vi "DL-SMART-MS-Modify-05-02 - 3.0.vi"() -> ()   [LabVIEW 2013]
uses:
  <vilib>/Utility/file.llb/Read From Spreadsheet File (DBL).vi
  <vilib>/vision/driver/NI_Vision_Acquisition_Software.lvlib
panel:
  out "Mass Spectrum (质谱图)":dbl[](graph)
  out "Image":T1(plugin-control)
  in  "Laser parameter":T3
  in  "ADC parameter":T4
  in  "ShutDownSystem":bool
  out "TenAccumulate":cluster{"MassX":dbl[], "TenScans":sgl[]}
  in  "ADC reference":refnum<vi>
  in  "set laser":bool
  in  "SetLaserEnergy":dbl(slide) min=0.0 max=50.0 scale=0.0..20.0
  in  "LaserHV":u8=50 min=1 max=100
  in  "LaserQuantity":u16
  in  "频率/Hz":u8=60
  out "plat zeroed":bool
  out "ADC aquiring":bool
  out "motor moving":bool
  out "busy":bool
  out "Pul.HV-Real":dbl
  in  "ReportResult":bool
  out "Identify Spcetrum":cluster{"all rows":dbl[], "all rows":dbl[]}[](graph)=[{"all rows"=array[50131 elements], "all rows"=array[50131 elements]}, {"all rows"=array[360 elements], "all rows"=[0.0, -15.85746, 0.0, 0.0, -4.11823, 0.0, 0.0, -20.55303, 0.0, 0.0, -3.65583, 0.0, 0.0, -2.69345, 0.0, 0.0, -4.4706, 0.0, 0.0, -6.07537, 0.0, 0.0, -4.25015, 0.0, 0.0, -6.95758, 0.0, 0.0, -2.04252, 0.0, 0.0, -7.70754, 0.0, 0.0, -4.28864, 0.0, 0.0, -4.00869, 0.0, 0.0, -4.47517, 0.0, 0.0, -14.21368, 0.0, 0.0, -6.66072, 0.0, 0.0, -6.50078, 0.0, 0.0, -3.75903, 0.0, 0.0, -17.29715, 0.0, 0.0, -6.92254, 0.0, 0.0, -2.52353, 0.0, 0.0, -3.06405, 0.0, 0.0, -16.54211, 0.0, 0.0, -5.10076, 0.0, 0.0, -8.01669, 0.0, 0.0, -40.71695, 0.0, 0.0, -4.03763, 0.0, 0.0, -3.14159, 0.0, 0.0, -2.79298, 0.0, 0.0, -13.41979, 0.0, 0.0, -7.6464, 0.0, 0.0, -6.18956, 0.0, 0.0, -2.44901, 0.0, 0.0, -5.1704, 0.0, 0.0, -3.62455, 0.0, 0.0, -6.443, 0.0, 0.0, -24.18432, 0.0, 0.0, -37.78631, 0.0, 0.0, -4.28528, 0.0, 0.0, -3.21654, 0.0, 0.0, -3.13522, 0.0, 0.0, -4.8477, 0.0, 0.0, -3.80614, 0.0, 0.0, -8.10386, 0.0, 0.0, -2.86382, 0.0, 0.0, -17.8978, 0.0, 0.0, -4.74503, 0.0, 0.0, -9.4855, 0.0, 0.0, -5.75364, 0.0, 0.0, -80.29859, 0.0, 0.0, -5.18928, 0.0, 0.0, -28.13783, 0.0, 0.0, -6.84449, 0.0, 0.0, -4.07742, 0.0, 0.0, -2.99391, 0.0, 0.0, -4.60838, 0.0, 0.0, -3.257, 0.0, 0.0, -5.79015, 0.0, 0.0, -24.98325, 0.0, 0.0, -4.30828, 0.0, 0.0, -5.54625, 0.0, 0.0, -5.47663, 0.0, 0.0, -100.0001, 0.0, 0.0, -21.11295, 0.0, 0.0, -12.03347, 0.0, 0.0, -6.35092, 0.0, 0.0, -4.71483, 0.0, 0.0, -6.58836, 0.0, 0.0, -3.41548, 0.0, 0.0, -3.10072, 0.0, 0.0, -4.79955, 0.0, 0.0, -4.88109, 0.0, 0.0, -32.02295, 0.0, 0.0, -20.17071, 0.0, 0.0, -9.63953, 0.0, 0.0, -8.63946, 0.0, 0.0, -6.018, 0.0, 0.0, -6.3389, 0.0, 0.0, -14.67808, 0.0, 0.0, -6.22948, 0.0, 0.0, -4.9166, 0.0, 0.0, -44.64096, 0.0, 0.0, -5.6163, 0.0, 0.0, -8.56872, 0.0, 0.0, -11.1186, 0.0, 0.0, -4.42493, 0.0, 0.0, -15.45284, 0.0, 0.0, -2.99091, 0.0, 0.0, -18.05376, 0.0, 0.0, -3.06669, 0.0, 0.0, -35.88844, 0.0, 0.0, -19.12645, 0.0, 0.0, -3.20878, 0.0, 0.0, -2.61247, 0.0, 0.0, -7.79975, 0.0, 0.0, -5.8874, 0.0, 0.0, -5.7487, 0.0, 0.0, -5.43834, 0.0, 0.0, -21.69908, 0.0, 0.0, -64.96584, 0.0, 0.0, -5.77762, 0.0, 0.0, -5.55465, 0.0, 0.0, -4.62119, 0.0, 0.0, -3.61176, 0.0, 0.0, -6.99332, 0.0, 0.0, -4.34549, 0.0, 0.0, -15.09003, 0.0, 0.0, -6.25437, 0.0, 0.0, -21.85243, 0.0, 0.0, -13.24381, 0.0, 0.0, -3.94672, 0.0, 0.0, -3.90192, 0.0, 0.0, -11.14967, 0.0, 0.0, -83.69183, 0.0, 0.0, -11.19559, 0.0, 0.0, -7.83445, 0.0, 0.0, -3.14763, 0.0, 0.0, -6.44728, 0.0, 0.0, -5.69155, 0.0, 0.0, -4.00216, 0.0]}]
  in  "IdentifyMS":bool
  in  "Identification Record (鉴定记录表)":i32(listbox)=6
  in  "Identification Results (单靶鉴定结果)":i32(listbox)=2
  in  "HVEnable":bool
  out "执行进度栏":u8(slide) caption="Vaccum" scale=0.0..1.0
  out "GateClose":bool
  out "LaserOK":bool
  out "HV-OK":bool
  out "Vacuum-OK":bool
  in  "Tab Control":T5(tab)
  in  "Shots":i32
  in  "EditAutoTar":bool
  in  "SinglePoint":bool
  in  "MultiPoints":bool
  in  "MultiTargets":bool
  in  "MCPHV-Set":dbl=1600.0 min=0.0 max=1600.0
  in  "LensHV-Set":dbl=8000.0 min=0.0 max=10000.0
  in  "Tar.HV-Set":dbl=18010.0 min=0.0 max=20000.0
  in  "Pul.HV-Set":dbl=1400.0 min=0.0 max=2000.0
  in  "PulseDelay":dbl
  in  "ADCFreq":dbl
  in  "CH1_Coupling":u64(ring)=2 items=["Volt DC"=1, "Volt AC"=2, "Ampere DC"=4, "Ampere AC"=8, "Ohm"=16]
  in  "Channel 1_Range":dbl(ring)=4.0 items=["80 V"=80.0, "40 V"=40.0, "20 V"=20.0, "8 V"=8.0, "4 V"=4.0, "2 V"=2.0, "800 mV"=0.8, "400 mV"=0.4, "200 mV"=0.2]
  in  "Anal. Setting File":string="High Mass"
  in  "SettingFileSave":bool caption="TakeMS"
  in  "SettingFileAppl":bool caption="TakeMS"
  in  "SettingDel":bool caption="TakeMS"
  in  "RunADC":bool caption="TakeMS"
  out "ADCstatus":bool
  in  "Vac_Prot.":bool
  in  "Turbo_Fore":bool
  in  "Main_Samp":bool
  in  "Samp_Atmos":bool
  in  "Fore_Samp":bool
  in  "StartPump":bool
  in  "SopPump":bool
  in  "Startsystem":bool
  out "TurboSpeed":dbl(knob) scale=0.0..100.0
  out "PumpKW":dbl
  out "PumpAmps":dbl
  out "PumpTemp":u16
  out "PumpVolts":dbl
  in  "laser OFF":bool
  in  "laser ON":bool
  out "cluster":T6
  in  "chamber in":bool caption="TakeMS"
  in  "GO":bool
  in  "Y":dbl min=0.0 max=55.0
  in  "X":dbl min=0.0 max=55.0
  in  "Y+":bool
  in  "Y-":bool
  in  "X-":bool
  in  "X+":bool
  in  "Plat_To_Zero":bool caption="TakeMS"
  in  "Plat_Cal":bool caption="TakeMS"
  out "Ty":dbl
  out "Tx":dbl
  out "Y当前":dbl
  out "X当前":dbl
  out "移动":bool
  out "Y满":bool
  out "Y标":bool
  out "X满":bool
  out "Y0":bool
  out "X0":bool
  out "靶位In/Out":bool
  out "仓门":bool
  out "Y过热":bool
  out "X过热":bool
  out "通讯":bool
  in  "chamber out":bool caption="TakeMS"
  in  "Operation Record":i32(listbox)
  in  "OptionRecordLoad 2":bool caption="TakeMS"
  in  "OptionRecordClear":bool caption="TakeMS"
  in  "OpenCloseGate":bool
  out "Tar.HV-Real":dbl
  out "LensHV-Real":dbl
  out "MCPHV-Real":dbl
  out "Lvaccum":dbl=0.83 format="%#_6e"
  out "Hvaccum":dbl=3.4e-05 format="%#_6e"
  in  "H12":bool
  in  "G12":bool
  in  "F12":bool
  in  "E12":bool
  in  "D12":bool
  in  "C12":bool
  in  "B12":bool
  in  "A12":bool
  in  "H11":bool
  in  "G11":bool
  in  "F11":bool
  in  "E11":bool
  in  "D11":bool
  in  "C11":bool
  in  "B11":bool
  in  "A11":bool
  in  "H10":bool
  in  "G10":bool
  in  "F10":bool
  in  "E10":bool
  in  "D10":bool
  in  "C10":bool
  in  "B10":bool
  in  "A10":bool
  in  "H9":bool
  in  "G9":bool
  in  "F9":bool
  in  "E9":bool
  in  "D9":bool
  in  "C9":bool
  in  "B9":bool
  in  "A9":bool
  in  "H8":bool
  in  "G8":bool
  in  "F8":bool
  in  "E8":bool
  in  "D8":bool
  in  "C8":bool
  in  "B8":bool
  in  "A8":bool
  in  "H7":bool
  in  "G7":bool
  in  "F7":bool
  in  "E7":bool
  in  "D7":bool
  in  "C7":bool
  in  "B7":bool
  in  "A7":bool
  in  "H6":bool
  in  "G6":bool
  in  "F6":bool
  in  "E6":bool
  in  "D6":bool
  in  "C6":bool
  in  "B6":bool
  in  "A6":bool
  in  "H5":bool
  in  "G5":bool
  in  "F5":bool
  in  "E5":bool
  in  "D5":bool
  in  "C5":bool
  in  "B5":bool
  in  "A5":bool
  in  "H4":bool
  in  "G4":bool
  in  "F4":bool
  in  "E4":bool
  in  "D4":bool
  in  "C4":bool
  in  "B4":bool
  in  "A4":bool
  in  "H3":bool
  in  "G3":bool
  in  "F3":bool
  in  "E3":bool
  in  "D3":bool
  in  "C3":bool
  in  "B3":bool
  in  "A3":bool
  in  "H2":bool
  in  "G2":bool
  in  "F2":bool
  in  "E2":bool
  in  "D2":bool
  in  "C2":bool
  in  "B2":bool
  in  "A2":bool
  in  "H1":bool
  in  "G1":bool
  in  "F1":bool
  in  "E1":bool
  in  "D1":bool
  in  "C1":bool
  in  "B1":bool
  in  "A1":bool
  in  "Clear":bool caption="TakeMS"
  in  "Add":bool caption="TakeMS"
  in  "TakeMS-Stop":bool caption="TakeMS"
  in  "TakeMS-Run":bool caption="TakeMS"
  # "Camera (摄像头)"
  # "Laser (激光)"
  # "Acq.(采谱)"
  # "1"
  # "2"
  # "3"
  # "4"
  # "5"
  # "6"
  # "7"
  # "8"
  # "9"
  # "10"
  # "11"
  # "12"
  # "Vacuum(真空)"
  # "A"
  # "Pa"
  # "High"
  # "B"
  # "Low"
  # "Pa"
  # "C"
  # "H.V.(高压)"
  # "D"
  # "Ident. (鉴定图)"
  # "MCP"
  # "V"
  # "E"
  # "Tar."
  # "V"
  # "F"
  # "Pul."
  # "V"
  # "G"
  # "Lens"
  # "V"
  # "H"
  # "Vauum (真空)"
  # "H.V. (高压)"
  # "Laser (激光)"
  # "Gate (仓门)"
  # "SinglePoint (单点)"
  # "MultiPoints (多点)"
  # "MultiTar. (多靶)"
  # "H.V. (高压参数)"
  # "ADC(采集卡设置)"
  # "ADCFreq(采样)"
  # "MCP (探测器)"
  # "V"
  # "Hz"
  # "Tar. (靶)"
  # "V"
  # "Setting File(设置文件)"
  # "Coupling"
  # "Pulse (脉冲)"
  # "V"
  # "IntRange"
  # "V"
  # "Lens (透镜)"
  # "Delay (延时)"
  # "ns"
  # "Turbo Pump"
  # "Sole. Valves"
  # "自锁保护"
  # "机械/分子"
  # "主仓/样仓"
  # "样仓/大气"
  # "机械/样仓"
  # "激光器状态"
  # "mm"
  # "mm"
  # "mm"
  # "mm"
  # "度"
  # "度"
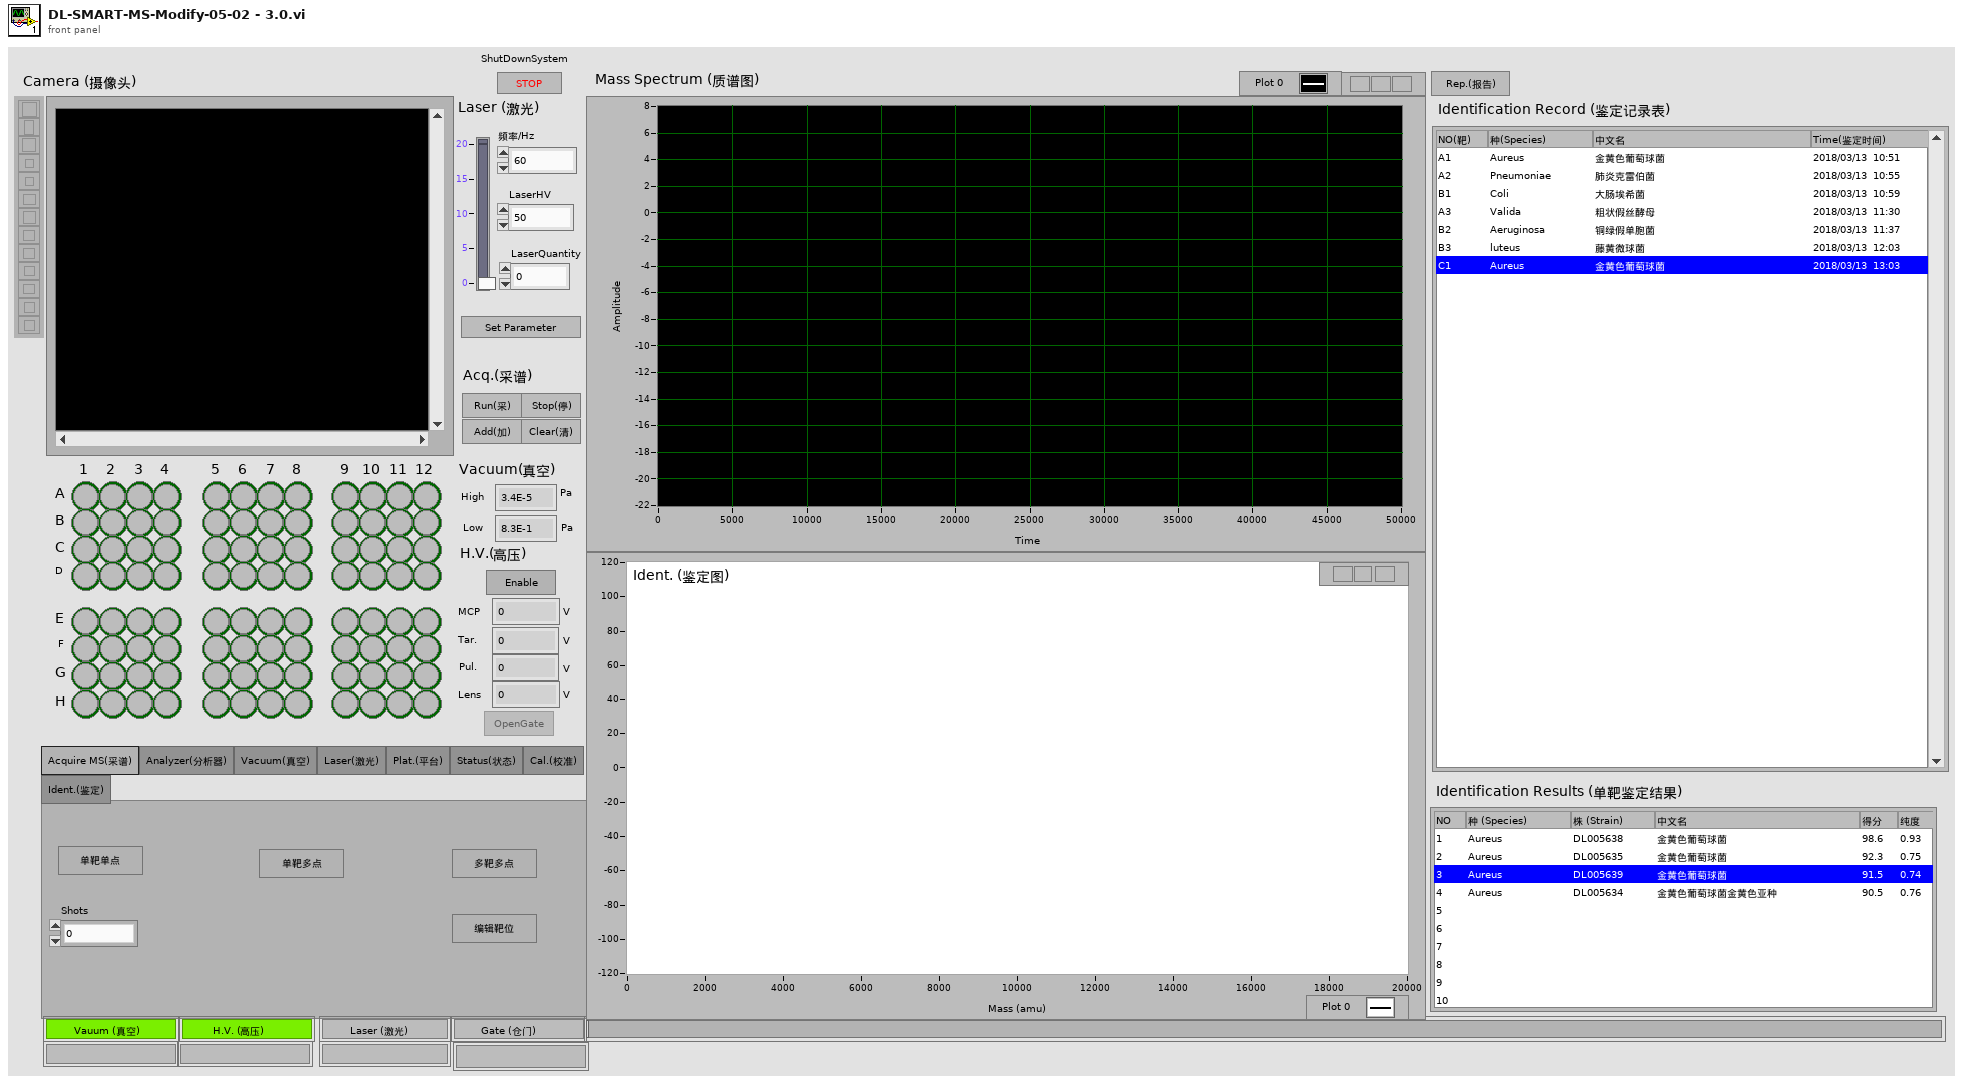
[diagram p1: front panel]
types:
  T1 = typedef "IMAQ Image.ctl" = refnum<image>
  T2 = typedef "Semaphore RefNum" = refnum<k1>
  T3 = cluster{"VISA resource name":refnum<visa-resource-name>, "standby":bool, "semaphore in":T2, "SetLaserEnergy":dbl}
  T4 = cluster{"TpDeviceHandle_t":u32, "Record Length/Samples":u64, "ShotsPerPoint":u16}
  T5 = enum32{"Acquire MS(采谱)", "Analyzer(分析器)", "Vacuum(真空)", "Laser(激光)", "Plat.(平台)", "Status(状态)", "Cal.(校准)", "Ident.(鉴定)"}
  T6 = cluster{"链接":bool, "待机":bool, "发射":bool, "[3]":bool, "内存":bool, "测能":bool, "温警":bool, "静态":bool, "操作":bool}
  T7 = cluster{"laser semaphore":T2, "pump semaphore":T2}
  T8 = enum8{"Enabled", "Disabled", "Disabled and Grayed Out"}
  T9 = cluster{"monitor":refnum<user-event>, "motor status":refnum<user-event>, "motor":refnum<user-event>, "notifier out":refnum<notifier>, "queue out":refnum<queue>, "AI":T2, "DI":T2, "CX":T2, "CY":T2}
  T10 = cluster{"AI Task":refnum<k21>, "AO Task":refnum<k21>, "DO Task":refnum<k21>, "DI Task":refnum<k21>, "PWM x":refnum<k21>, "PWM y":refnum<k21>, "counter x":refnum<k21>, "counter y":refnum<k21>}
  T11 = cluster{"tasks":cluster{"AI Task":refnum<k21>, "AO Task":refnum<k21>, "DO Task":refnum<k21>, "DI Task":refnum<k21>, "PWM x":refnum<k21>, "PWM y":refnum<k21>, "counter x":refnum<k21>, "counter y":refnum<k21>}, "interface":cluster{"monitor":refnum<user-event>, "motor status":refnum<user-event>, "motor":refnum<user-event>, "notifier out":refnum<notifier>, "queue out":refnum<queue>, "AI":T2, "DI":T2, "CX":T2, "CY":T2}, "error out":errorcluster}
  T12 = cluster{"ConfiguredPumpCom":refnum<visa-resource-name>, "ConfiguredLaserCom":refnum<visa-resource-name>}
  T13 = cluster{"Type":u32, "Version":u32, "Flags":u32, "SerialNumberHigh":u32, "SerialNumberLow":u32, "BusType":u32, "InterfaceName":string, "VendorName":string, "ModelName":string, "CameraFileName":string, "CameraAttributeURL":string}[]
  T14 = cluster{"Type":u32, "Version":u32, "Flags":u32, "SerialNumberHigh":u32, "SerialNumberLow":u32, "BusType":u32, "InterfaceName":string, "VendorName":string, "ModelName":string, "CameraFileName":string, "CameraAttributeURL":string}
  T15 = typedef "IMAQdx.ctl" = refnum<k21>
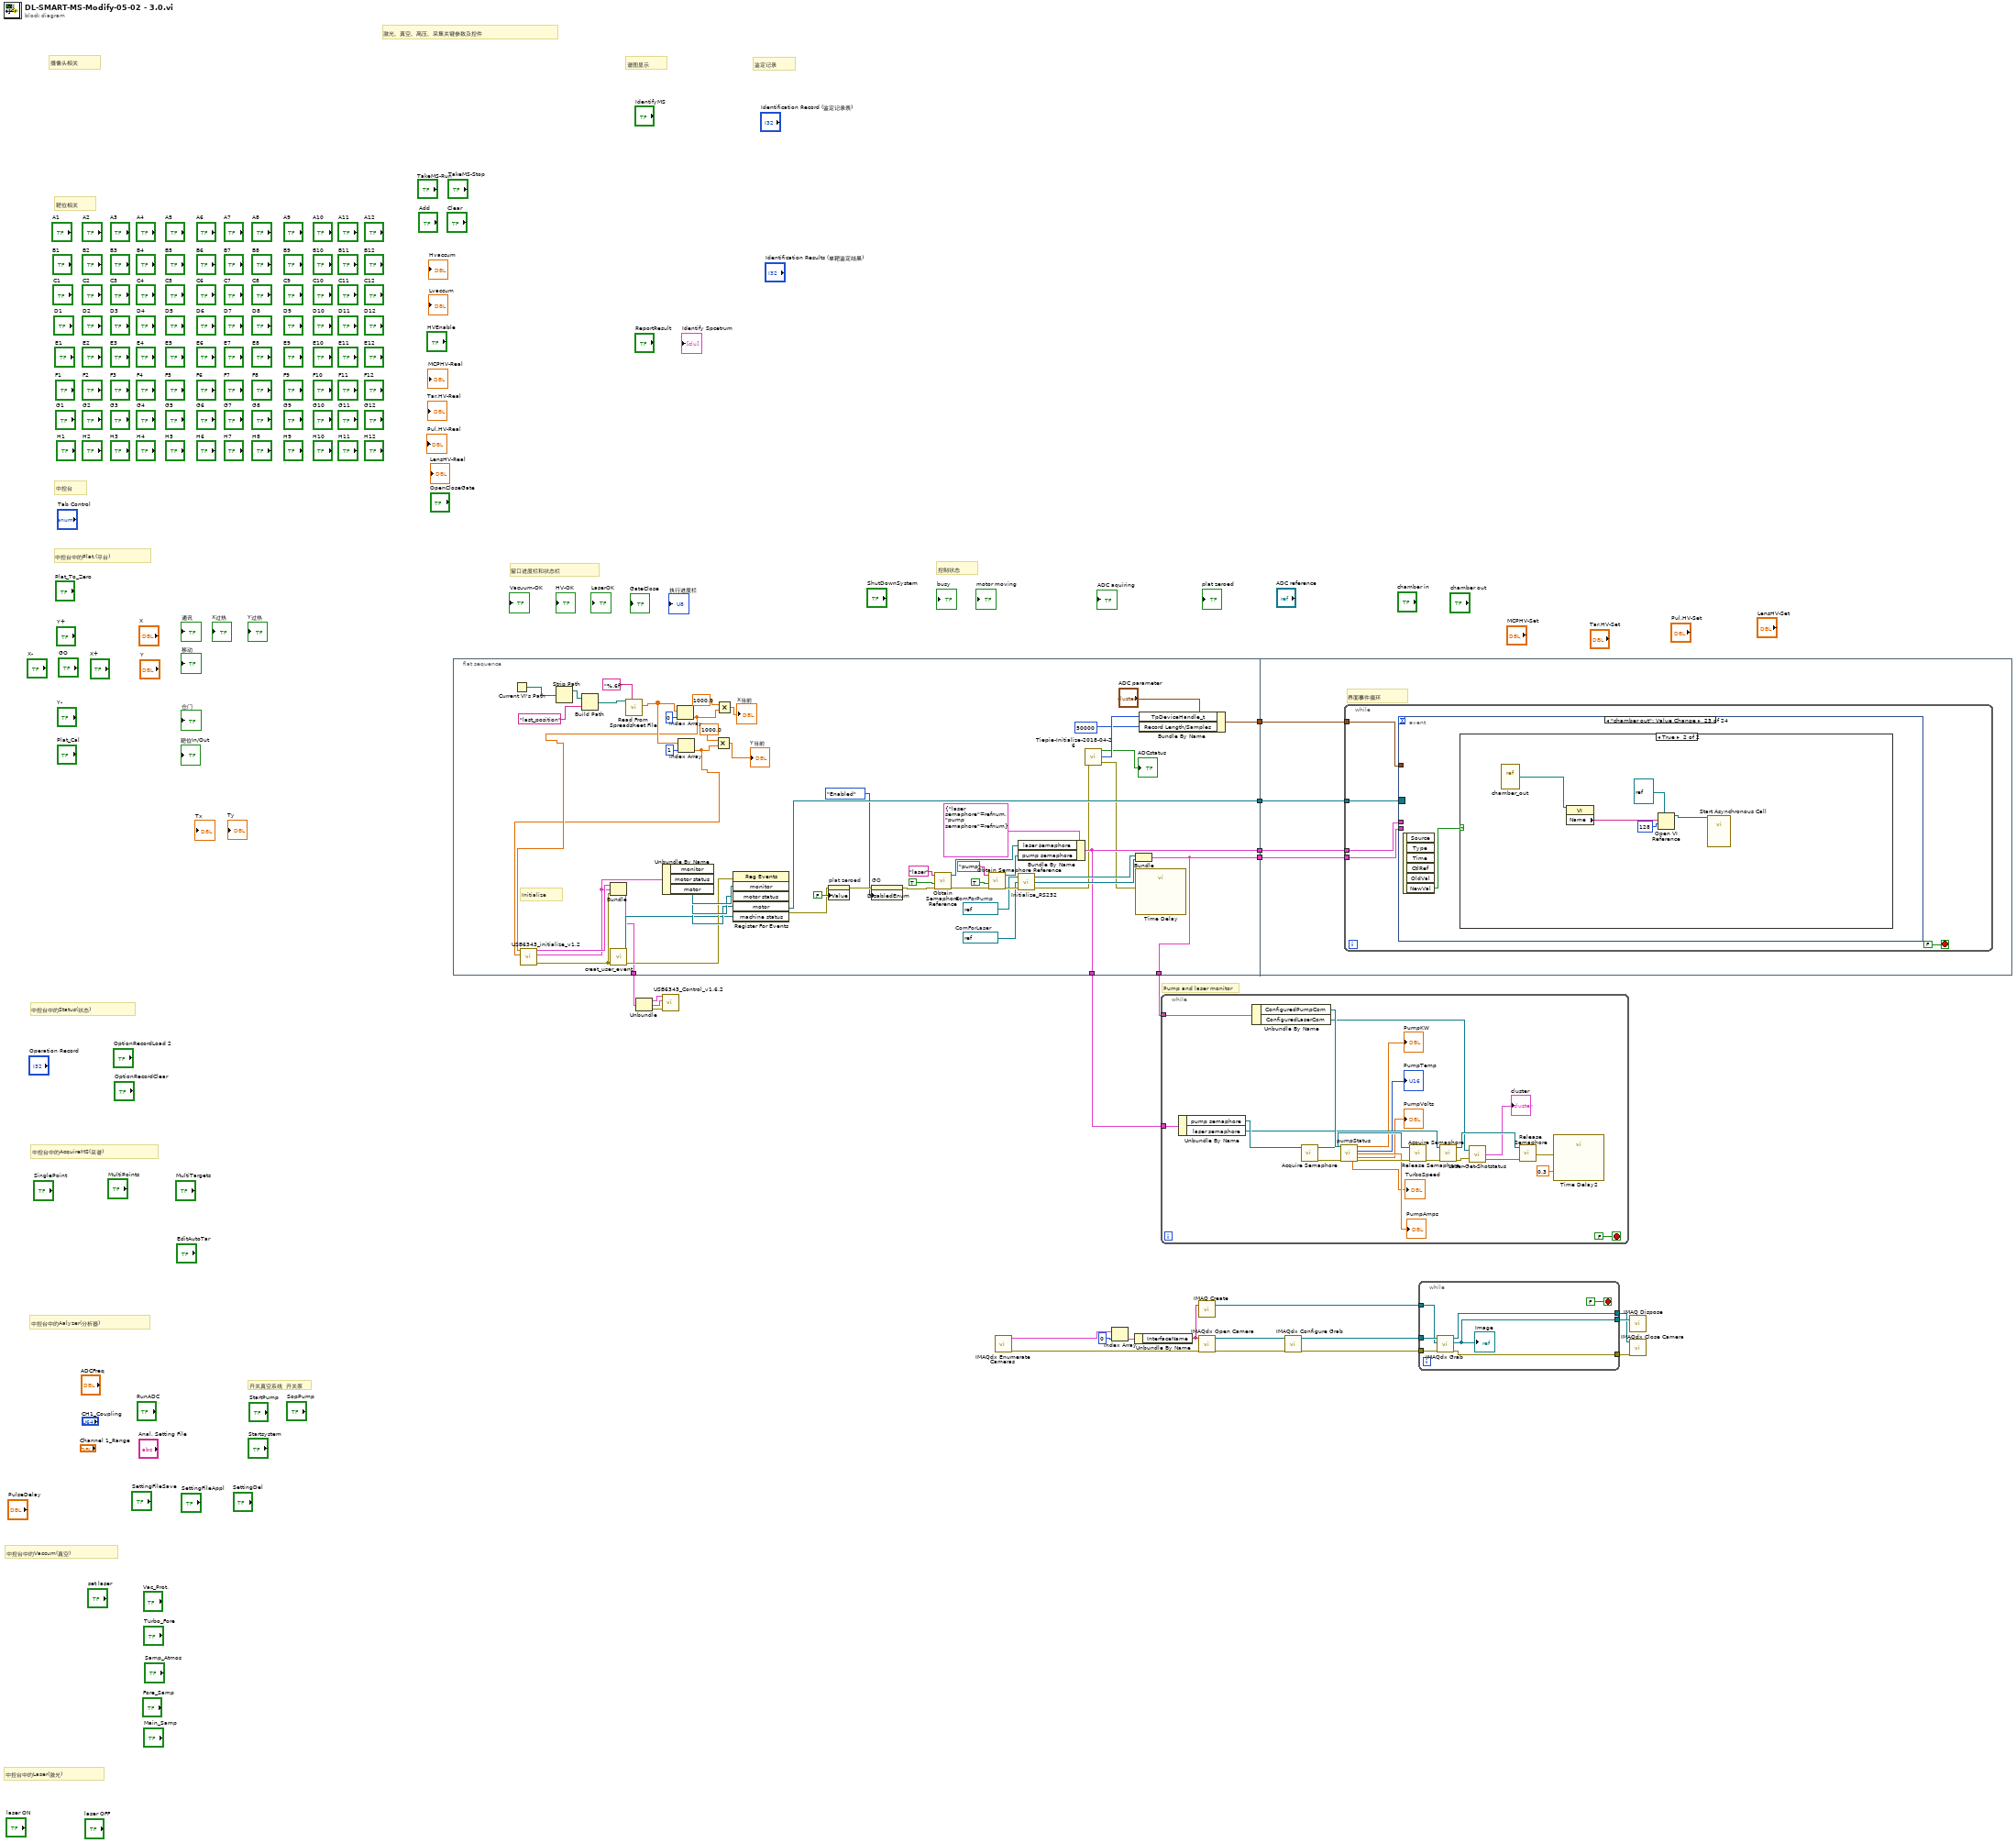
[diagram p0: block diagram]
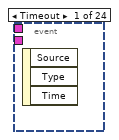
[diagram p2: hidden frame]
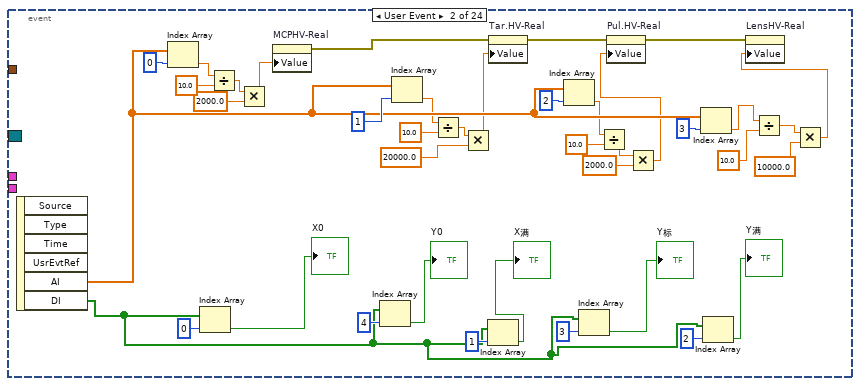
[diagram p3: hidden frame]
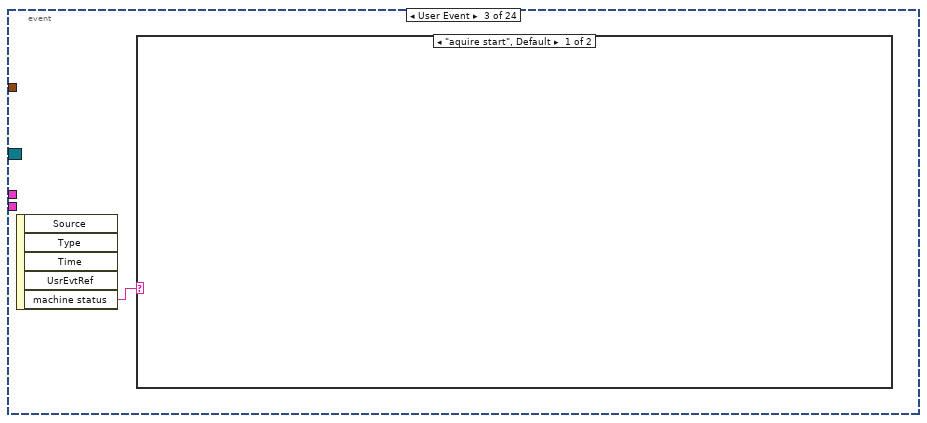
[diagram p4: hidden frame]
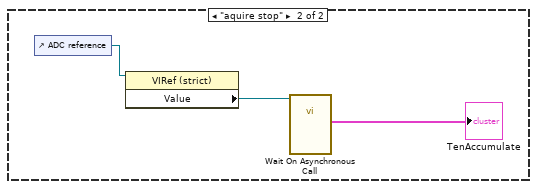
[diagram p5: hidden frame]
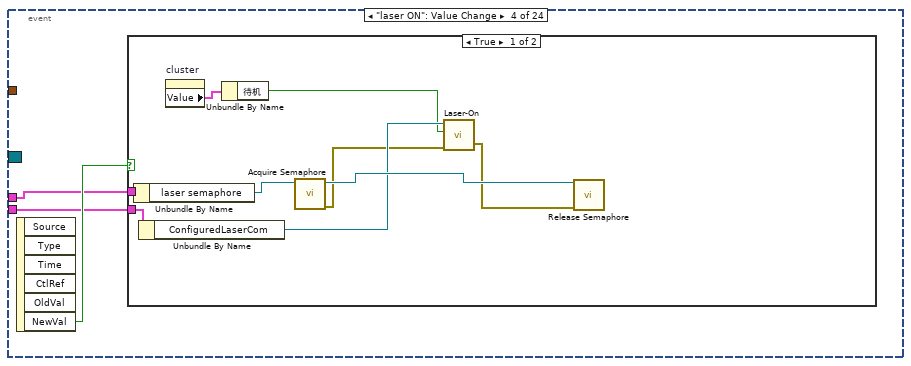
[diagram p6: hidden frame]
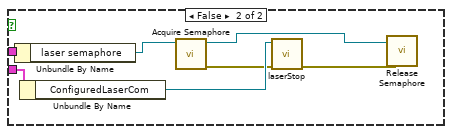
[diagram p7: hidden frame]
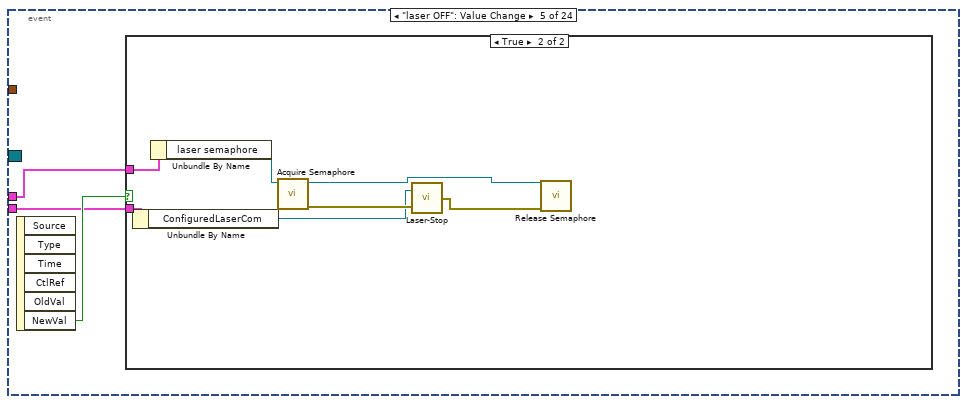
[diagram p8: hidden frame]
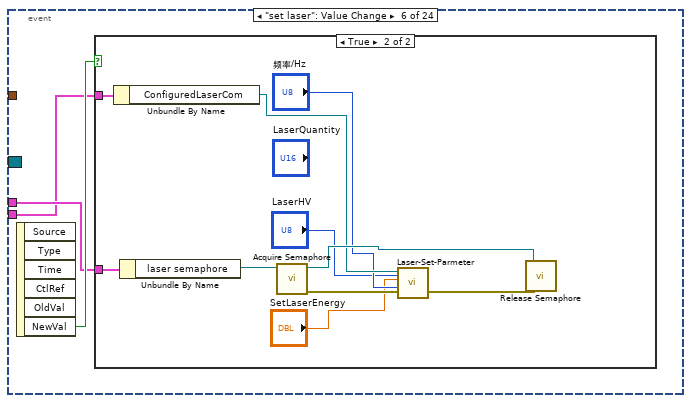
[diagram p10: hidden frame]
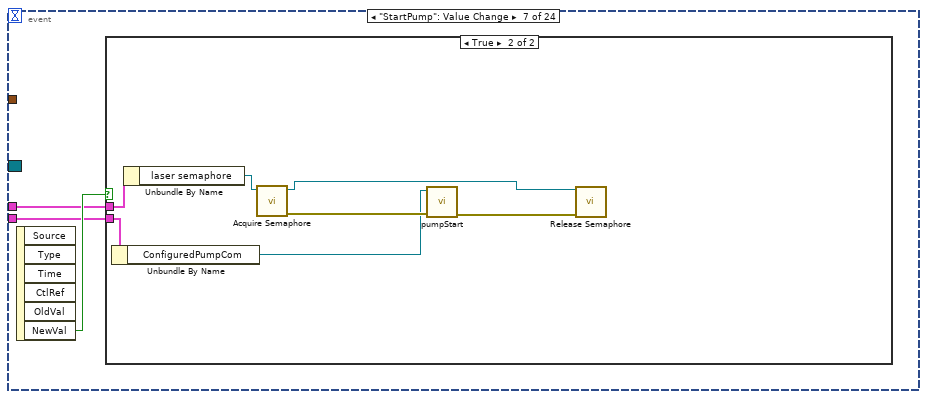
[diagram p12: hidden frame]
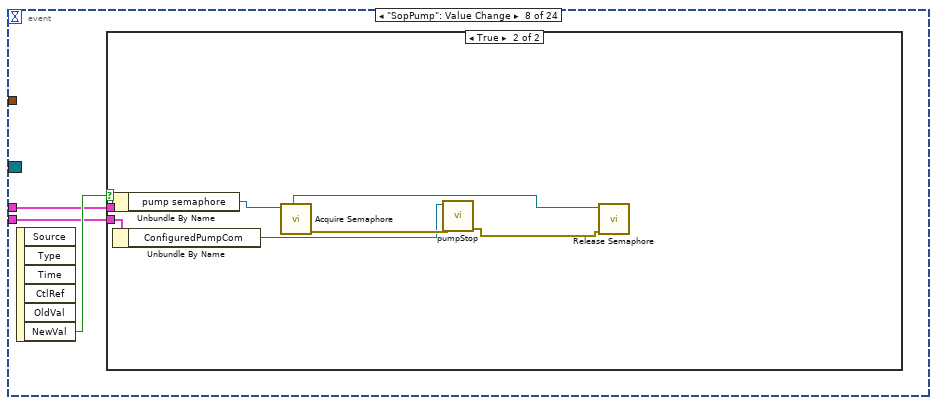
[diagram p14: hidden frame]
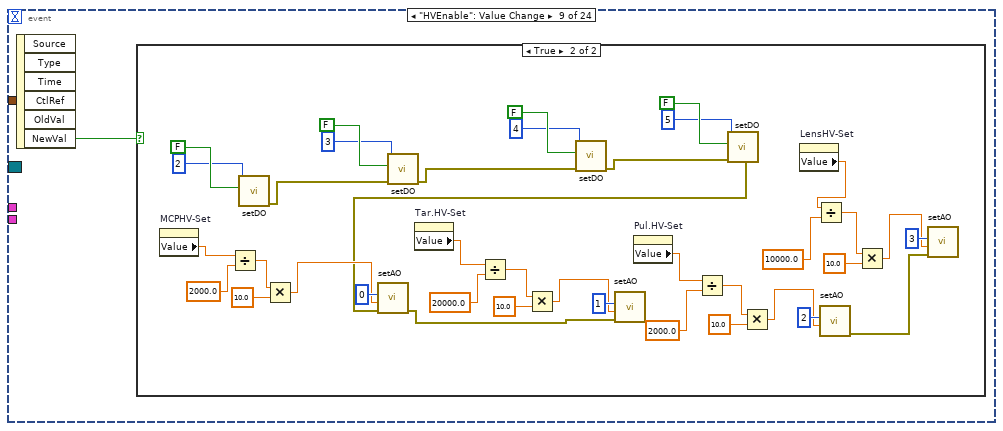
[diagram p16: hidden frame]
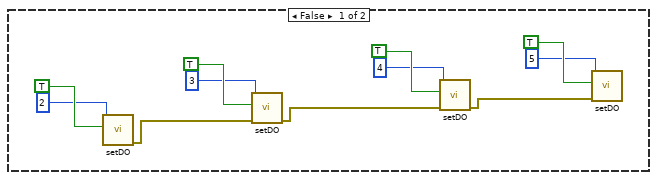
[diagram p17: hidden frame]
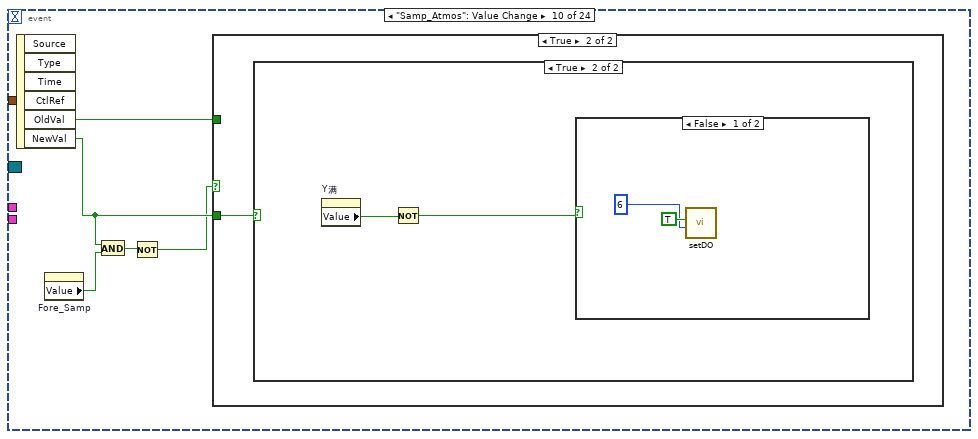
[diagram p18: hidden frame]
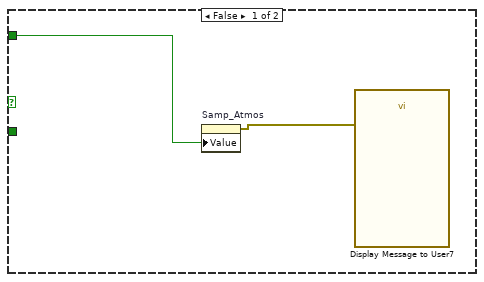
[diagram p19: hidden frame]
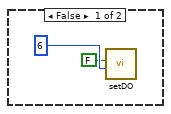
[diagram p20: hidden frame]
diagram:
  # "Pump and laser monitor"
  # "开关真空系统  开关泵"
  # "控制状态"
  # "鉴定记录"
  # "谱图显示"
  # "激光、真空、高压、采集关键参数及控件"
  # "窗口进度栏和状态栏"
  # "中控台中的Laser(激光)"
  # "中控台中的Vaccum(真空)"
  # "中控台中的Aalyzer(分析器)"
  # "中控台中的AcquireMS(采谱)"
  # "中控台中的Status(状态)"
  # "中控台中的Plat.(平台)"
  # "中控台"
  # "靶位相关"
  # "摄像头相关"
  n1 = flat-sequence {
    tunnel: [w71] -> w23
    tunnel: [w48] -> w22
    tunnel: [w48] -> w20
    tunnel: [w47] -> w21
    tunnel: [w47] -> w19
    tunnel: [w51] -> w18
    tunnel: [w39] -> w14
    tunnel: w23 -> [w78]
    tunnel: w22 -> [w77]
    tunnel: w21 -> [w76]
    tunnel: w14 -> [w75]
    frame #0 {
      w45 = refnum<visa-resource-name> "COM3"  # ComForLaser
      w46 = refnum<visa-resource-name> "COM4"  # ComForPump
      # "Initialize"
      n2 = Current VI's Path() -> (path=w37:path)
      n3 = Strip Path(path=w37) -> (stripped path=w36:path)  [unwired: 1 out]
      n4 = Build Path(base path=w36, name or relative path="last_position") -> (appended path=w34:path)
      n5 = call-poly <vilib>:"Read From Spreadsheet File.vi"("format (%.3f)"="%.6f", "file path (dialog if empty)"=w34) -> ("first row"=w32:dbl[])  [unwired: 5 in, 4 out]
      n6 = Index Array(array=w32, index=0) -> (element=w29:dbl)
      n7 = Index Array(array=w32, index=1) -> (element=w26:dbl)
      n8 = call "USB6343_initialize_v1.2.vi"("Y initial position"=w26, "X initial position"=w29) -> ("error out"=w52:errorcluster, "interface"=w53:T9, "tasks"=w54:T10)  [unwired: 7 in]
      n9 = Bundle("tasks"=w54, "interface"=w53, "error out"=w52) -> (w51:T11)  [unwired: 1 in]
      n10 = call "creat_user_event.vi"("error in (no error)"=w52) -> ("error out"=w65:errorcluster, "machine status"=w62:refnum<user-event>)  [unwired: 9 in]
      n11 = Unbundle By Name(w53) -> ("monitor"=w74:refnum<user-event>, "motor status"=w73:refnum<user-event>, "motor"=w72:refnum<user-event>)
      n12 = Multiply(x=1000.0, y=w26) -> (x*y=→"Y当前":dbl)
      n13 = Multiply(x=1000.0, y=w29) -> (x*y=→"X当前":dbl)
      n14 = register-events(error in=w65, w74, w73, w72, w62) -> (reference out=w71:refnum<event-registration>, error out=w64:errorcluster)  [unwired: 1 in]
      n15 = property on="plat zeroed" class="Bool (strict)"(error in=w64, "Value"=FALSE ("plat zeroed")) -> (error out=w69:errorcluster)  [unwired: 1 in, 1 out]
      n16 = property on="GO" class="Bool (strict)"(error in=w69, "DisabledEnum"=T8."Enabled" ("Disabled")) -> (error out=w63:errorcluster)  [unwired: 1 in, 1 out]
      n17 = call <vilib>:"Obtain Semaphore Reference.vi"("error in (no error)"=w63, "create if not found (T)"=TRUE, "name (unnamed)"="laser") -> ("error out"=w58:errorcluster, "semaphore"=w55:T2)  [unwired: 2 in, 1 out]
      n18 = call <vilib>:"Obtain Semaphore Reference.vi"("error in (no error)"=w58, "create if not found (T)"=TRUE, "name (unnamed)"="pump") -> ("error out"=w57:errorcluster, "semaphore"=w49:T2)  [unwired: 2 in, 1 out]
      n19 = Bundle By Name(cluster=T7 {"laser semaphore"=refnum, "pump semaphore"=refnum}, "laser semaphore"=w55, "pump semaphore"=w49) -> (w48:T7)
      n20 = call "Initialize_RS232.vi"("error in (no error)"=w57, "ComForLaser"=w45, "ComForPump"=w46) -> ("error out"=w44:errorcluster, "ConfiguredLaserCom"=w60:refnum<visa-resource-name>, "ConfiguredPumpCom"=w61:refnum<visa-resource-name>)
      n21 = call "Tiepie-Initialize-2018-04-26.vi"("error in (no error)"=w44) -> ("error out"=w43:errorcluster, "TpDeviceHandle_t"=w41:u32, "Card-OK"=→"ADCstatus":bool)  [unwired: 3 in]
      n22 = Bundle("ConfiguredPumpCom"=w61, "ConfiguredLaserCom"=w60) -> (w47:T12)  [unwired: 1 in]
      n23 = call "Time Delay"("error in (no error)"=w43) -> ()  [unwired: 10 in, 1 out]
      n24 = Bundle By Name(cluster="ADC parameter", "TpDeviceHandle_t"=w41, "Record Length/Samples"=u64 50000) -> (w39:T4)
    }
    frame #1 {
      # "界面事件循环"
      n25 = while {
        tunnel: w78 -> [w83]
        tunnel: w76 -> [w82]
        tunnel: w77 -> [w81]
        tunnel: w75 -> [w79]
        stop <- FALSE stop-if-true
        n26 = event shown="[22] \"chamber out\": Value Change" {
          selector: w83 -> [_ _ _ _ _ _ _ _ _ _ _ _ _ _ _ _ _ _ _ _ _ _ _ _]
          dyn-events: _ -> [_ _ _ _ _ _ _ _ _ _ _ _ _ _ _ _ _ _ _ _ _ _ _ _]
          timeout: _ -> [_ _ _ _ _ _ _ _ _ _ _ _ _ _ _ _ _ _ _ _ _ _ _ _]
          tunnel: w82 -> [_ _ _ w127 w146 w156 w169 w179 _ _ _ _ _ _ _ _ _ w307 _ _ _ _ _ w357]
          tunnel: w81 -> [_ _ _ w128 w147 w157 w170 w180 _ _ _ _ _ _ _ _ _ w308 _ _ _ _ _ _]
          tunnel: w79 -> [_ _ _ _ _ _ _ _ _ _ _ _ _ _ _ _ _ w309 _ _ _ _ _ _]
          event Timeout {
            n27 = event-data() -> ()  [unwired: 1 in, 3 out]
          }
          event User Event {
            n28 = event-data() -> ("AI"=w115:dbl[], "DI"=w105:bool[])  [unwired: 1 in, 4 out]
            n29 = Index Array(array=w115, index=0) -> (element=w103:dbl)
            n30 = Index Array(array=w105, index=0) -> (element=→"X0":bool)
            n31 = Divide(x=w103, y=10.0) -> (x/y=w101:dbl)
            n32 = Multiply(x=w101, y=2000.0) -> (x*y=w99:dbl)
            n33 = property on="MCPHV-Real" class="DigNum (strict)"("Value"=w99) -> (error out=w122:errorcluster)  [unwired: 2 in, 1 out]
            n34 = Index Array(array=w105, index=4) -> (element=→"Y0":bool)
            n35 = Index Array(array=w115, index=1) -> (element=w98:dbl)
            n36 = Divide(x=w98, y=10.0) -> (x/y=w96:dbl)
            n37 = Multiply(x=w96, y=20000.0) -> (x*y=w94:dbl)
            n38 = Index Array(array=w105, index=1) -> (element=→"X满":bool)
            n39 = property on="Tar.HV-Real" class="DigNum (strict)"(error in=w122, "Value"=w94) -> (error out=w121:errorcluster)  [unwired: 1 in, 1 out]
            n40 = Index Array(array=w115, index=2) -> (element=w93:dbl)
            n41 = Index Array(array=w105, index=3) -> (element=→"Y标":bool)
            n42 = Divide(x=w93, y=10.0) -> (x/y=w91:dbl)
            n43 = Multiply(x=w91, y=2000.0) -> (x*y=w89:dbl)
            n44 = property on="Pul.HV-Real" class="DigNum (strict)"(error in=w121, "Value"=w89) -> (error out=w120:errorcluster)  [unwired: 1 in, 1 out]
            n45 = Index Array(array=w115, index=3) -> (element=w88:dbl)
            n46 = Index Array(array=w105, index=2) -> (element=→"Y满":bool)
            n47 = Divide(x=w88, y=10.0) -> (x/y=w86:dbl)
            n48 = Multiply(x=w86, y=10000.0) -> (x*y=w84:dbl)
            n49 = property on="LensHV-Real" class="DigNum (strict)"(error in=w120, "Value"=w84) -> ()  [unwired: 1 in, 2 out]
          }
          event User Event {
            n50 = event-data() -> ("machine status"=w123:string)  [unwired: 1 in, 4 out]
            n51 = case shown="\"aquire start\", Default" w123 {
              frame "aquire start", Default {
              }
              frame "aquire stop" {
                n52 = control-ref of="ADC reference"() -> (w126:refnum<vi>)
                n53 = property class="VIRef (strict)"(reference=w126) -> ("Value"=w125:refnum<vi>)  [unwired: 1 in, 2 out]
                n54 = call-by-ref "Wait On Asynchronous Call"(reference=w125) -> ("TenAccumulate"=→"TenAccumulate":cluster{"MassX":dbl[], "TenScans":sgl[]})  [unwired: 12 in, 2 out]
              }
            }
          }
          event "laser ON": Value Change {
            n55 = event-data() -> ("NewVal"=w129:bool)  [unwired: 1 in, 5 out]
            n56 = case shown="True" w129 {
              tunnel: w128 -> [w138 w145]
              tunnel: w127 -> [w136 w143]
              frame True {
                n57 = Unbundle By Name(w138) -> ("laser semaphore"=w137:T2)
                n58 = Unbundle By Name(w136) -> ("ConfiguredLaserCom"=w133:refnum<visa-resource-name>)
                n59 = property on="cluster" class="Clust (strict)"() -> ("Value"=w134:T6)  [unwired: 2 in, 2 out]
                n60 = Unbundle By Name(w134) -> ("待机"=w130:bool)
                n61 = call <vilib>:"Acquire Semaphore.vi"("semaphore"=w137) -> ("error out"=w132:errorcluster, "semaphore out"=w135:T2)  [unwired: 4 in, 1 out]
                n62 = call "Laser-On.vi"("error in (no error)"=w132, "standby"=w130, "VISA resource name"=w133) -> ("error out"=w131:errorcluster)  [unwired: 1 in, 1 out]
                n63 = call <vilib>:"Release Semaphore.vi"("error in (no error)"=w131, "semaphore"=w135) -> ()  [unwired: 4 in, 2 out]
              }
              frame False {
                n64 = Unbundle By Name(w145) -> ("laser semaphore"=w144:T2)
                n65 = Unbundle By Name(w143) -> ("ConfiguredLaserCom"=w142:refnum<visa-resource-name>)
                n66 = call <vilib>:"Acquire Semaphore.vi"("semaphore"=w144) -> ("error out"=w141:errorcluster, "semaphore out"=w139:T2)  [unwired: 4 in, 1 out]
                n67 = call "laserStop.vi"("error in (no error)"=w141, "VISA resource name"=w142) -> ("error out"=w140:errorcluster)  [unwired: 9 in]
                n68 = call <vilib>:"Release Semaphore.vi"("error in (no error)"=w140, "semaphore"=w139) -> ()  [unwired: 4 in, 2 out]
              }
            }
          }
          event "laser OFF": Value Change {
            n69 = event-data() -> ("NewVal"=w148:bool)  [unwired: 1 in, 5 out]
            n70 = case shown="True" w148 {
              tunnel: w147 -> [_ w155]
              tunnel: w146 -> [_ w152]
              frame False {
              }
              frame True {
                n71 = Unbundle By Name(w152) -> ("ConfiguredLaserCom"=w151:refnum<visa-resource-name>)
                n72 = Unbundle By Name(w155) -> ("laser semaphore"=w154:T2)
                n73 = call <vilib>:"Acquire Semaphore.vi"("semaphore"=w154) -> ("error out"=w153:errorcluster, "semaphore out"=w149:T2)  [unwired: 4 in, 1 out]
                n74 = call "Laser-Stop.vi"("error in (no error)"=w153, "VISA resource name"=w151) -> ("error out"=w150:errorcluster)
                n75 = call <vilib>:"Release Semaphore.vi"("error in (no error)"=w150, "semaphore"=w149) -> ()  [unwired: 4 in, 2 out]
              }
            }
          }
          event "set laser": Value Change {
            n76 = event-data() -> ("NewVal"=w158:bool)  [unwired: 1 in, 5 out]
            n77 = case shown="True" w158 {
              tunnel: w157 -> [_ w168]
              tunnel: w156 -> [_ w164]
              frame False {
              }
              frame True {
                n78 = Unbundle By Name(w164) -> ("ConfiguredLaserCom"=w163:refnum<visa-resource-name>)
                n79 = Unbundle By Name(w168) -> ("laser semaphore"=w167:T2)
                n80 = call <vilib>:"Acquire Semaphore.vi"("semaphore"=w167) -> ("error out"=w165:errorcluster, "semaphore out"=w166:T2)  [unwired: 4 in, 1 out]
                n81 = call "Laser-Set-Parmeter.vi"("error in (no error)"=w165, "LaserHV"="LaserHV", "LaserFreq"="频率/Hz", "SetLaserEnergy"="SetLaserEnergy", "VISA resource name"=w163) -> ("error out"=w160:errorcluster)  [unwired: 1 in, 1 out]
                n82 = call <vilib>:"Release Semaphore.vi"("error in (no error)"=w160, "semaphore"=w166) -> ()  [unwired: 4 in, 2 out]
              }
            }
          }
          event "StartPump": Value Change {
            n83 = event-data() -> ("NewVal"=w171:bool)  [unwired: 1 in, 5 out]
            n84 = case shown="True" w171 {
              tunnel: w170 -> [_ w176]
              tunnel: w169 -> [_ w175]
              frame False {
              }
              frame True {
                n85 = Unbundle By Name(w175) -> ("ConfiguredPumpCom"=w174:refnum<visa-resource-name>)
                n86 = Unbundle By Name(w176) -> ("laser semaphore"=w173:T2)
                n87 = call <vilib>:"Acquire Semaphore.vi"("semaphore"=w173) -> ("error out"=w178:errorcluster, "semaphore out"=w172:T2)  [unwired: 4 in, 1 out]
                n88 = call "pumpStart.vi"("error in (no error)"=w178, "VISA resource name"=w174) -> ("error out"=w177:errorcluster)  [unwired: 9 in]
                n89 = call <vilib>:"Release Semaphore.vi"("error in (no error)"=w177, "semaphore"=w172) -> ()  [unwired: 4 in, 2 out]
              }
            }
          }
          event "SopPump": Value Change {
            n90 = event-data() -> ("NewVal"=w181:bool)  [unwired: 1 in, 5 out]
            n91 = case shown="True" w181 {
              tunnel: w180 -> [_ w185]
              tunnel: w179 -> [_ w183]
              frame False {
              }
              frame True {
                n92 = Unbundle By Name(w185) -> ("pump semaphore"=w184:T2)
                n93 = Unbundle By Name(w183) -> ("ConfiguredPumpCom"=w182:refnum<visa-resource-name>)
                n94 = call <vilib>:"Acquire Semaphore.vi"("semaphore"=w184) -> ("error out"=w188:errorcluster, "semaphore out"=w186:T2)  [unwired: 4 in, 1 out]
                n95 = call "pumpStop.vi"("error in (no error)"=w188, "VISA resource name"=w182) -> ("error out"=w187:errorcluster)  [unwired: 9 in]
                n96 = call <vilib>:"Release Semaphore.vi"("error in (no error)"=w187, "semaphore"=w186) -> ()  [unwired: 4 in, 2 out]
              }
            }
          }
          event "HVEnable": Value Change {
            n97 = event-data() -> ("NewVal"=w189:bool)  [unwired: 1 in, 5 out]
            n98 = case shown="True" w189 {
              frame False {
                n99 = call "setDO.vi"("channel"=2, "on/off"=TRUE) -> ("错误输出"=w192:errorcluster)  [unwired: 9 in]
                n100 = call "setDO.vi"("错误输入（无错误）"=w192, "channel"=3, "on/off"=TRUE) -> ("错误输出"=w191:errorcluster)  [unwired: 8 in]
                n101 = call "setDO.vi"("错误输入（无错误）"=w191, "channel"=4, "on/off"=TRUE) -> ("错误输出"=w190:errorcluster)  [unwired: 8 in]
                n102 = call "setDO.vi"("错误输入（无错误）"=w190, "channel"=5, "on/off"=TRUE) -> ()  [unwired: 8 in, 1 out]
              }
              frame True {
                n103 = property on="MCPHV-Set" class="DigNum (strict)"() -> ("Value"=w222:dbl)  [unwired: 2 in, 2 out]
                n104 = Divide(x=w222, y=2000.0) -> (x/y=w225:dbl)
                n105 = call "setDO.vi"("channel"=2, "on/off"=FALSE) -> ("错误输出"=w230:errorcluster)  [unwired: 9 in]
                n106 = Multiply(x=w225, y=10.0) -> (x*y=w223:dbl)
                n107 = call "setDO.vi"("错误输入（无错误）"=w230, "channel"=3, "on/off"=FALSE) -> ("错误输出"=w229:errorcluster)  [unwired: 8 in]
                n108 = property on="Tar.HV-Set" class="DigNum (strict)"() -> ("Value"=w216:dbl)  [unwired: 2 in, 2 out]
                n109 = Divide(x=w216, y=20000.0) -> (x/y=w219:dbl)
                n110 = Multiply(x=w219, y=10.0) -> (x*y=w217:dbl)
                n111 = call "setDO.vi"("错误输入（无错误）"=w229, "channel"=4, "on/off"=FALSE) -> ("错误输出"=w228:errorcluster)  [unwired: 8 in]
                n112 = property on="Pul.HV-Set" class="DigNum (strict)"() -> ("Value"=w208:dbl)  [unwired: 2 in, 2 out]
                n113 = Divide(x=w208, y=2000.0) -> (x/y=w211:dbl)
                n114 = call "setDO.vi"("错误输入（无错误）"=w228, "channel"=5, "on/off"=FALSE) -> ("错误输出"=w214:errorcluster)  [unwired: 8 in]
                n115 = call "setAO.vi"("错误输入（无错误）"=w214, "value"=w223, "channel"=0) -> ("错误输出"=w215:errorcluster)  [unwired: 8 in]
                n116 = call "setAO.vi"("错误输入（无错误）"=w215, "value"=w217, "channel"=1) -> ()  [unwired: 8 in, 1 out]
                n117 = Multiply(x=w211, y=10.0) -> (x*y=w209:dbl)
                n118 = property on="LensHV-Set" class="DigNum (strict)"() -> ("Value"=w201:dbl)  [unwired: 2 in, 2 out]
                n119 = Divide(x=w201, y=10000.0) -> (x/y=w205:dbl)
                n120 = call "setAO.vi"("value"=w209, "channel"=2) -> ("错误输出"=w202:errorcluster)  [unwired: 9 in]
                n121 = Multiply(x=w205, y=10.0) -> (x*y=w204:dbl)
                n122 = call "setAO.vi"("错误输入（无错误）"=w202, "value"=w204, "channel"=3) -> ()  [unwired: 8 in, 1 out]
              }
            }
          }
          event "Samp_Atmos": Value Change {
            n123 = event-data() -> ("OldVal"=w239:bool, "NewVal"=w243:bool)  [unwired: 1 in, 4 out]
            n124 = property on="Fore_Samp" class="Bool (strict)"() -> ("Value"=w242:bool)  [unwired: 2 in, 2 out]
            n125 = And(x=w243, y=w242) -> (x .and. y?=w241:bool)
            n126 = Not(x=w241) -> (.not. x?=w240:bool)
            n127 = case shown="True" w240 {
              tunnel: w243 -> [_ w246]
              tunnel: w239 -> [w245 _]
              frame False {
                n128 = property on="Samp_Atmos" class="Bool (strict)"("Value"=w245) -> (error out=w244:errorcluster)  [unwired: 2 in, 1 out]
                n129 = call "Display Message to User7"("error in (no error)"=w244) -> ()  [unwired: 9 in, 2 out]
              }
              frame True {
                n130 = case shown="True" w246 {
                  frame False {
                    n131 = call "setDO.vi"("channel"=6, "on/off"=FALSE) -> ()  [unwired: 9 in, 1 out]
                  }
                  frame True {
                    n132 = property on="Y满" class="Bool (strict)"() -> ("Value"=w250:bool)  [unwired: 2 in, 2 out]
                    n133 = Not(x=w250) -> (.not. x?=w249:bool)
                    n134 = case shown="False" w249 {
                      frame False {
                        n135 = call "setDO.vi"("channel"=6, "on/off"=TRUE) -> ()  [unwired: 9 in, 1 out]
                      }
                      frame True {
                        n136 = call "Display Message to User6"() -> ()  [unwired: 10 in, 2 out]
                      }
                    }
                  }
                }
              }
            }
          }
          event "Fore_Samp": Value Change {
            n137 = event-data() -> ("OldVal"=w253:bool, "NewVal"=w257:bool)  [unwired: 1 in, 4 out]
            n138 = property on="Samp_Atmos" class="Bool (strict)"() -> ("Value"=w256:bool)  [unwired: 2 in, 2 out]
            n139 = And(x=w257, y=w256) -> (x .and. y?=w255:bool)
            n140 = Not(x=w255) -> (.not. x?=w254:bool)
            n141 = case shown="True" w254 {
              tunnel: w257 -> [_ w260]
              tunnel: w253 -> [w259 _]
              frame False {
                n142 = property on="Fore_Samp" class="Bool (strict)"("Value"=w259) -> (error out=w258:errorcluster)  [unwired: 2 in, 1 out]
                n143 = call "Display Message to User8"("error in (no error)"=w258) -> ()  [unwired: 9 in, 2 out]
              }
              frame True {
                n144 = case shown="True" w260 {
                  frame False {
                    n145 = call "setDO.vi"("channel"=7, "on/off"=FALSE) -> ()  [unwired: 9 in, 1 out]
                  }
                  frame True {
                    n146 = property on="Y满" class="Bool (strict)"() -> ("Value"=w264:bool)  [unwired: 2 in, 2 out]
                    n147 = Not(x=w264) -> (.not. x?=w263:bool)
                    n148 = case shown="False" w263 {
                      frame False {
                        n149 = call "setDO.vi"("channel"=7, "on/off"=TRUE) -> ()  [unwired: 9 in, 1 out]
                      }
                      frame True {
                        n150 = call "Display Message to User"() -> ()  [unwired: 10 in, 2 out]
                      }
                    }
                  }
                }
              }
            }
          }
          event "MCPHV-Set": Value Change {
            n151 = event-data() -> ("NewVal"=w272:dbl)  [unwired: 1 in, 5 out]
            n152 = Divide(x=w272, y=2000.0) -> (x/y=w269:dbl)
            n153 = Multiply(x=w269, y=10.0) -> (x*y=w267:dbl)
            n154 = call "setAO.vi"("value"=w267, "channel"=0) -> ()  [unwired: 9 in, 1 out]
          }
          event "Tar.HV-Set": Value Change {
            n155 = event-data() -> ("NewVal"=w278:dbl)  [unwired: 1 in, 5 out]
            n156 = Divide(x=w278, y=20000.0) -> (x/y=w275:dbl)
            n157 = Multiply(x=w275, y=10.0) -> (x*y=w273:dbl)
            n158 = call "setAO.vi"("value"=w273, "channel"=1) -> ()  [unwired: 9 in, 1 out]
          }
          event "Pul.HV-Set": Value Change {
            n159 = event-data() -> ("NewVal"=w284:dbl)  [unwired: 1 in, 5 out]
            n160 = Divide(x=w284, y=2000.0) -> (x/y=w281:dbl)
            n161 = Multiply(x=w281, y=10.0) -> (x*y=w279:dbl)
            n162 = call "setAO.vi"("value"=w279, "channel"=2) -> ()  [unwired: 9 in, 1 out]
          }
          event "LensHV-Set": Value Change {
            n163 = event-data() -> ("NewVal"=w290:dbl)  [unwired: 1 in, 5 out]
            n164 = Divide(x=w290, y=10000.0) -> (x/y=w287:dbl)
            n165 = Multiply(x=w287, y=10.0) -> (x*y=w286:dbl)
            n166 = call "setAO.vi"("value"=w286, "channel"=3) -> ()  [unwired: 9 in, 1 out]
          }
          event User Event {
            n167 = event-data() -> ("status"=w291:string)  [unwired: 1 in, 5 out]
            n168 = case shown="\"stop\", Default" w291 {
              frame "stop", Default {
                n169 = property on="GO" class="Bool (strict)"("DisabledEnum"=T8."Enabled" ("Disabled")) -> (error out=w294:errorcluster)  [unwired: 2 in, 1 out]
                n170 = property on="移动" class="Bool (strict)"(error in=w294, "Value"=FALSE ("移动")) -> (error out=w292:errorcluster)  [unwired: 1 in, 1 out]
                n171 = call "record_position.vi"("错误输入（无错误）"=w292) -> ()  [unwired: 10 in, 1 out]
              }
              frame "moving" {
                n172 = property on="GO" class="Bool (strict)"("DisabledEnum"=T8."Disabled and Grayed Out" ("Disabled")) -> (error out=w297:errorcluster)  [unwired: 2 in, 1 out]
                n173 = property on="移动" class="Bool (strict)"(error in=w297, "Value"=TRUE ("移动")) -> ()  [unwired: 1 in, 2 out]
              }
            }
          }
          event User Event {
            n174 = event-data() -> ("source"=w300:string, "value"=w299:dbl)  [unwired: 1 in, 4 out]
            n175 = case shown="\"Y\", Default" w300 {
              tunnel: w299 -> [w303 w306]
              frame "Y", Default {
                n176 = Multiply(x=w303, y=1000.0) -> (x*y=w301:dbl)
                n177 = property on="Y当前" class="DigNum (strict)"("Value"=w301) -> ()  [unwired: 2 in, 2 out]
              }
              frame "X" {
                n178 = Multiply(x=w306, y=1000.0) -> (x*y=w304:dbl)
                n179 = property on="X当前" class="DigNum (strict)"("Value"=w304) -> ()  [unwired: 2 in, 2 out]
              }
            }
          }
          event "SinglePoint": Value Change {
            n180 = event-data() -> ("NewVal"=w310:bool)  [unwired: 1 in, 5 out]
            n181 = case shown="True" w310 {
              tunnel: w309 -> [_ w323]
              tunnel: w308 -> [_ w320]
              tunnel: w307 -> [_ w319]
              frame False {
              }
              frame True {
                n182 = Unbundle By Name(w319) -> ("ConfiguredLaserCom"=w316:refnum<visa-resource-name>)
                n183 = Unbundle By Name(w320) -> ("laser semaphore"=w314:T2)
                n184 = property on="cluster" class="Clust (strict)"() -> ("Value"=w318:T6)  [unwired: 2 in, 2 out]
                n185 = Bundle By Name(cluster=w323, "ShotsPerPoint"="Shots") -> (w321:T4)
                n186 = Unbundle By Name(w318) -> ("待机"=w315:bool)
                n187 = property on="SetLaserEnergy" class="Slide (strict)"() -> ("Value"=w313:dbl)  [unwired: 2 in, 2 out]
                n188 = Bundle By Name(cluster="Laser parameter", "VISA resource name"=w316, "standby"=w315, "semaphore in"=w314, "SetLaserEnergy"=w313) -> (w312:T3)
                n189 = call "Tiepie-takeData-2018-04-26.vi"("ADC parameter"=w321, "Laser parameter"=w312) -> ("Array out"=→"Mass Spectrum (质谱图)":dbl[])  [unwired: 2 in, 1 out]
              }
            }
          }
          event "Plat_To_Zero": Value Change {
            n190 = event-data() -> ("NewVal"=w330:bool)  [unwired: 1 in, 5 out]
            n191 = property on="OpenCloseGate" class="Bool"("DisabledEnum"=T8."Disabled and Grayed Out" ("Disabled")) -> (error out=w329:errorcluster)  [unwired: 2 in, 1 out]
            n192 = case shown="True" w330 {
              tunnel: w329 -> [w331 w333]
              tunnel: [w331 w332] -> w326
              frame False {
              }
              frame True {
                n193 = call "plate_cal.vi"("错误输入（无错误）"=w333) -> ("错误输出"=w332:errorcluster)  [unwired: 10 in]
              }
            }
            n194 = property on="plat zeroed" class="Bool (strict)"(error in=w326, "Value"=TRUE ("plat zeroed")) -> (error out=w324:errorcluster)  [unwired: 1 in, 1 out]
            n195 = property on="GO" class="Bool (strict)"(error in=w324, "DisabledEnum"=T8."Enabled" ("Disabled")) -> ()  [unwired: 1 in, 2 out]
          }
          event "GO": Value Change {
            n196 = event-data() -> ("NewVal"=w334:bool)  [unwired: 1 in, 5 out]
            n197 = case shown="True" w334 {
              frame False {
              }
              frame True {
                n198 = property on="X" class="DigNum (strict)"() -> (error out=w339:errorcluster, "Value"=w337:dbl)  [unwired: 2 in, 1 out]
                n199 = property on="Y" class="DigNum (strict)"(error in=w339) -> (error out=w338:errorcluster, "Value"=w336:dbl)  [unwired: 1 in, 1 out]
                n200 = vi-ref "goto.vi"() -> (w343:refnum<vi>)
                n201 = property class="VI"(reference=w343, error in=w338) -> ("Name"=w342:string)  [unwired: 2 out]
                n202 = Open VI Reference(type specifier VI Refnum (for type only)=refnum<vi> refnum, vi path=w342, options=128) -> (vi reference=w340:refnum<vi>)  [unwired: 3 in, 1 out]
                n203 = call-by-ref "Start Asynchronous Call"(reference=w340, "Y(mm)"=w336, "X(mm)"=w337) -> ()  [unwired: 10 in, 3 out]
              }
            }
          }
          event "X+": Value Change {
            n204 = event-data() -> ("NewVal"=w344:bool)  [unwired: 1 in, 5 out]
            n205 = case shown="True" w344 {
              frame False {
              }
              frame True {
              }
            }
          }
          event "chamber in": Value Change {
            n206 = event-data() -> ("NewVal"=w345:bool)  [unwired: 1 in, 5 out]
            n207 = case shown="True" w345 {
              frame False {
              }
              frame True {
                n208 = vi-ref "chamber_in.vi"() -> (w348:refnum<vi>)
                n209 = property class="VI"(reference=w348) -> ("Name"=w350:string)  [unwired: 1 in, 2 out]
                n210 = Open VI Reference(type specifier VI Refnum (for type only)=refnum<vi> refnum, vi path=w350, options=128) -> (vi reference=w346:refnum<vi>)  [unwired: 3 in, 1 out]
                n211 = call-by-ref "Start Asynchronous Call"(reference=w346) -> ()  [unwired: 13 in, 2 out]
              }
            }
          }
          event "chamber out": Value Change {
            n212 = event-data() -> ("NewVal"=w351:bool)  [unwired: 1 in, 5 out]
            n213 = case shown="True" w351 {
              frame False {
              }
              frame True {
                n214 = vi-ref "chamber_out.vi"() -> (w353:refnum<vi>)
                n215 = property class="VI"(reference=w353) -> ("Name"=w356:string)  [unwired: 1 in, 2 out]
                n216 = Open VI Reference(type specifier VI Refnum (for type only)=refnum<vi> refnum, vi path=w356, options=128) -> (vi reference=w354:refnum<vi>)  [unwired: 3 in, 1 out]
                n217 = call-by-ref "Start Asynchronous Call"(reference=w354) -> ()  [unwired: 13 in, 2 out]
              }
            }
          }
          event "ShutDownSystem": Value Change {
            n218 = event-data() -> ("NewVal"=w358:bool)  [unwired: 1 in, 5 out]
            n219 = case shown="True" w358 {
              tunnel: w357 -> [_ w362]
              frame False {
              }
              frame True {
                n220 = Unbundle By Name(w362) -> ("ConfiguredPumpCom"=w361:refnum<visa-resource-name>, "ConfiguredLaserCom"=w360:refnum<visa-resource-name>)
                n221 = VISA Close(VISA resource name=w361) -> (error out=w359:errorcluster)  [unwired: 1 in]
                n222 = VISA Close(VISA resource name=w360, error in (no error)=w359) -> ()  [unwired: 1 out]
              }
            }
          }
        }
      }
    }
  }
  n223 = Unbundle(w18) -> ("tasks"=w17:T10, "interface"=w16:T9, "error out"=w15:errorcluster)
  n224 = call "USB6343_Control_v1.6.2.vi"("error in"=w15, "interface"=w16, "tasks"=w17) -> ()  [unwired: 9 in]
  n225 = call <vilib>:"IMAQdx Enumerate Cameras.vi"() -> ("error out"=w4:errorcluster, "Camera Information Array"=w1:T13)  [unwired: 10 in]
  n226 = Index Array(array=w1, index=0) -> (element=w3:T14)
  n227 = Unbundle By Name(w3) -> ("InterfaceName"=w12:string)
  n228 = while {
    tunnel: w20 -> [w384]
    tunnel: w19 -> [w382]
    stop <- FALSE stop-if-true
    n229 = Unbundle By Name(w384) -> ("pump semaphore"=w383:T2, "laser semaphore"=w376:T2)
    n230 = Unbundle By Name(w382) -> ("ConfiguredPumpCom"=w381:refnum<visa-resource-name>, "ConfiguredLaserCom"=w367:refnum<visa-resource-name>)
    n231 = call <vilib>:"Acquire Semaphore.vi"("semaphore"=w383) -> ("error out"=w380:errorcluster, "semaphore out"=w378:T2)  [unwired: 4 in, 1 out]
    n232 = call "pumpStatus.vi"("VISA resource name"=w381, "error in (no error)"=w380) -> ("PumpKW"=→"PumpKW":dbl, "PumpTemp"=→"PumpTemp":u16, "PumpAmps"=→"PumpAmps":dbl, "PumpVolts"=→"PumpVolts":dbl, "TurboSpeed"=→"TurboSpeed":dbl, "error out"=w379:errorcluster)  [unwired: 8 in]
    n233 = call <vilib>:"Release Semaphore.vi"("error in (no error)"=w379, "semaphore"=w378) -> ("error out"=w377:errorcluster)  [unwired: 4 in, 1 out]
    n234 = call <vilib>:"Acquire Semaphore.vi"("error in (no error)"=w377, "semaphore"=w376) -> ("error out"=w366:errorcluster, "semaphore out"=w375:T2)  [unwired: 3 in, 1 out]
    n235 = call "Laser-Get-Shotstatus.vi"("VISA resource name"=w367, "error in (no error)"=w366) -> ("cluster"=→"cluster":T6, "error out"=w365:errorcluster)  [unwired: 1 out]
    n236 = call <vilib>:"Release Semaphore.vi"("error in (no error)"=w365, "semaphore"=w375) -> ("error out"=w374:errorcluster)  [unwired: 4 in, 1 out]
    n237 = call "Time Delay2"("error in (no error)"=w374, "Delay Time (s)"=0.3) -> ()  [unwired: 9 in, 1 out]
  }
  n238 = call "IMAQ Create"("Image Name"=w12) -> ("New Image"=w6:T1)  [unwired: 4 in, 1 out]
  n239 = call <vilib>:"IMAQdx Open Camera.vi"("error in"=w4, "Session In"=w12) -> ("error out"=w11:errorcluster, "Session Out"=w13:T15)  [unwired: 8 in]
  n240 = call <vilib>:"IMAQdx Configure Grab.vi"("error in"=w11, "Session In"=w13) -> ("error out"=w10:errorcluster, "Session Out"=w5:T15)  [unwired: 8 in]
  n241 = while {
    tunnel: w10 -> [w391]
    tunnel: w5 -> [w390]
    tunnel: w6 -> [w389]
    tunnel: [w388] -> w7
    tunnel: [w387] -> w8
    tunnel: [w386] -> w9
    stop <- FALSE stop-if-true
    n242 = call <vilib>:"IMAQdx Grab.vi"("error in"=w391, "Image In"=w389, "Session In"=w390) -> ("error out"=w388:errorcluster, "Image Out"=w386:T1, "Session Out"=w387:T15)  [unwired: 5 in, 1 out]
    "Image" <- w386
  }
  n243 = call "IMAQ Dispose"("Image"=w9) -> ()  [unwired: 5 in, 1 out]
  n244 = call <vilib>:"IMAQdx Close Camera.vi"("error in"=w7, "Session In"=w8) -> ()  [unwired: 9 in, 1 out]
